vi "Do Core.vi"(8 "error in (no error)":errorcluster, 9 "Actor in":refnum<class "Actor.lvclass">, 11 "Reply Message":refnum<class "Iterate Reply Msg.lvclass">) -> (0 "error out":errorcluster, 1 "Actor out":refnum<class "Actor.lvclass">, 2 "Reply":bool=TRUE)   [LabVIEW 2021, in "Example Actor.lvlib" / "Iterate Reply Msg.lvclass"]
doc: "(<B>Filename</B>: Actor Framework.lvlib:Reply Msg.lvclass:Do Core.vi)\n\nDefines what an actor does when it receives <B>Reply Message</B>. This method also defines the <B>Reply</B> that is returned to the actor that sent <B>Reply Message</B>.\n\nBy default, this method does nothing, and <B>Reply</B> is the ancestor Message class. A child class must override this method to define behavior and specify a child of the Message class to return in the <B>Reply</B> output."
uses:
  Iterate Reply Msg.lvclass
  <vilib>/ActorFramework/Actor/Actor.lvclass
  Example Actor/Example Actor.lvclass
  C:/Program Files/National Instruments/LabVIEW 2021/vi.lib/ActorFramework/Actor/Actor.lvclass
  Iterate Reply Msg.lvclass/Iterate Reply Msg.ctl
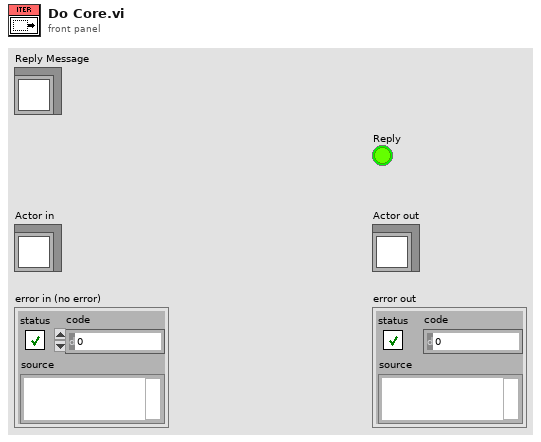
[diagram p1: front panel]
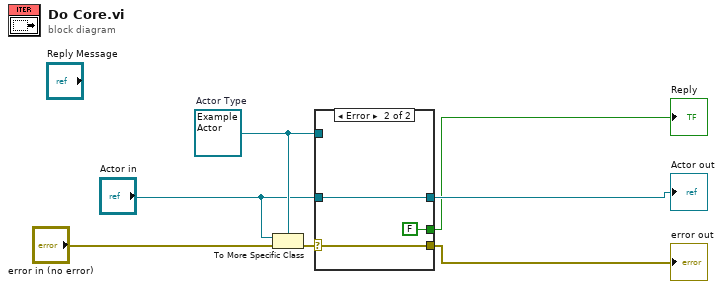
[diagram p0: block diagram]
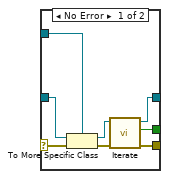
[diagram p2: hidden frame]
diagram:
  w6 = refnum<class "Example Actor.lvclass"> refnum  # Actor Type
  n1 = To More Specific Class(target class=w6, reference="Actor in", error in="error in (no error)") -> (error out=w7:errorcluster)  [unwired: 1 out]
  n2 = case shown="Error" w7 {
    selector: w7 -> [w15 w18]
    tunnel: [w10 w18] -> w3
    tunnel: [w9 w17] -> w2
    tunnel: "Actor in" -> [w14 w17]
    tunnel: w6 -> [w13 _]
    tunnel: [w8 FALSE ("Continue")] -> w1
    frame No Error {
      n3 = To More Specific Class ("Actor Cast")(target class=w13, reference=w14, error in=w15) -> (specific class reference=w12:refnum<class "Example Actor.lvclass">, error out=w11:errorcluster)
      n4 = call "Iterate.vi"("error in (no error)"=w11, "Example Actor in"=w12) -> ("error out"=w10:errorcluster, "Continue"=w8:bool, "Example Actor out"=w9:refnum<class "Example Actor.lvclass">)  [unwired: 7 in]
    }
    frame Error {
    }
  }
  "error out" <- w3
  "Actor out" <- w2
  "Reply" <- w1
